vi "PIPBOY_Dlg_MainUi.vi"(11 "Path":path) -> ()   [LabVIEW 2014]
uses:
  PIPBOY_Ctl_Td_PaletteItem.ctl
  <vilib>/picture/picture.llb/imagedata.ctl
  <userlib>/_saphir_lib_vbx.llb/XXX_Tlk_Tree-GetItemPosition_Scalar__saphir_lib_vbx.vi
  <userlib>/_saphir_lib_vbx.llb/XXX_Tlk_Tree-Cleanup_Scalar__saphir_lib_vbx.vi
  <userlib>/_saphir_lib_vbx.llb/XXX_Tlk_Tree-AddElement_Scalar__saphir_lib_vbx.vi
panel:
  in  "ListRemove":bool
  in  "ListAdd":bool
  out "Item Icon":picture
  in  "Item Name":string
  in  "Item Function":i32(ring) items=["<Palette>"=-1, "Complex To Re/Im"=0, "Complex To Polar"=1, "Re/Im To Complex"=2, "Polar To Complex"=3, "Complex Conjugate"=4, "Sign"=5, "Add"=6, "Subtract"=7, "Multiply"=8, "Divide"=9, "Absolute Value"=10, "Round To Nearest"=11, "Quotient & Remainder"=12, "Increment"=13, "Decrement"=14, "Reciprocal"=15, "Square Root"=16, "And"=17, "Or"=18, "Exclusive Or"=19, "Not"=20, "Negate"=21, "Random Number (0-1)"=22, "Not And"=23, "Not Or"=24, "Not Exclusive Or"=25, "Scale By Power Of 2"=26, "Round Toward -Infinity"=27, "Round Toward +Infinity"=28, "Path To String"=29, "String To Path"=30, "Cast Unit Bases"=31, "Implies"=32, "Logical Shift"=33, "Rotate"=34, "First Call?"=35, "DataSocket Open"=36, "DataSocket Close"=37, "DataSocket Read"=38, "DataSocket Write"=39, "Equal?"=40, "Greater Or Equal?"=41, "Less Or Equal?"=42, "Not Equal?"=43, "Max & Min"=44, "Greater?"=45, "Less?"=46, "Empty String/Path?"=47, "Equal To 0?"=48, "Greater Or Equal To 0?"=49, "Less Or Equal To 0?"=50, "Not Equal To 0?"=51, "Greater Than 0?"=52, "Less Than 0?"=53, "Decimal Digit?"=54, "Sort 1D Array"=55, "Hex Digit?"=56, "Printable?"=57, "White Space?"=58, "Lexical Class"=59, "In Range and Coerce"=60, "Not A Number/Path/Refnum?"=61, "Octal Digit?"=62, "To Byte Integer"=63, "To Word Integer"=64, "To Long Integer"=65, "To Unsigned Byte Integer"=66, "To Unsigned Word Integer"=67, "To Unsigned Long Integer"=68, "To Single Precision Float"=69, "To Double Precision Float"=70, "To Extended Precision Float"=71, "Mantissa & Exponent"=72, "To Single Precision Complex"=73, "To Double Precision Complex"=74, "To Extended Precision Complex"=75, "To Quad Integer"=76, "To Unsigned Quad Integer"=77, "Flatten To String"=78, "Unflatten From String"=79, "Swap Bytes"=80, "Swap Words"=81, "Type Cast"=82, "Boolean To (0,1)"=83, "Array To Cluster"=84, "Cluster To Array"=85, "Split Number"=86, "Join Numbers"=87, "Number To Decimal String"=88, "Number To Hexadecimal String"=89, "Number To Octal String"=90, "Number To Engineering String"=91, "Decimal String To Number"=92, "Hexadecimal String To Number"=93, "Octal String To Number"=94, "Fract/Exp String To Number"=95, "To Upper Case"=96, "To Lower Case"=97, "Sine"=98, "Cosine"=99, "Tangent"=100, "Secant"=101, "Cosecant"=102, "Cotangent"=103, "Inverse Sine"=104, "Inverse Cosine"=105, "Inverse Tangent"=106, "Natural Logarithm"=107, "Logarithm Base 10"=108, "Exponential"=109, "Power Of 10"=110, "Power Of X"=111, "Hyperbolic Sine"=112, "Hyperbolic Cosine"=113, "Hyperbolic Tangent"=114, "Inverse Hyperbolic Sine"=115, "Inverse Hyperbolic Cosine"=116, "Inverse Hyperbolic Tangent"=117, "Sine & Cosine"=118, "Natural Logarithm (Arg +1)"=119, "Exponential (Arg) -1"=120, "Power Of 2"=121, "Logarithm Base X"=122, "Logarithm Base 2"=123, "Sinc"=124, "Inverse Tangent (2 Input)"=125, "Tick Count (ms)"=126, "Wait (ms)"=127, "Get Date/Time In Seconds"=128, "Date/Time To Seconds"=129, "Seconds To Date/Time"=130, "Wait Until Next ms Multiple"=131, "Wait For Front Panel Activity"=132, "Generate Front Panel Activity"=133, "One Button Dialog"=134, "Two Button Dialog"=135, "Stop"=136, "Quit LabVIEW"=137, "Control Help Window"=138, "Get Help Window Status"=139, "Control Online Help"=140, "New Directory"=141, "Open File"=142, "New File"=143, "Close File (deprecated)"=144, "Flush File (deprecated)"=145, "Read File"=146, "Write File"=147, "Seek"=148, "EOF"=149, "Lock Range"=150, "Access Rights"=151, "File/Directory Info (deprecated)"=152, "Volume Info"=153, "Move (deprecated)"=154, "Copy (deprecated)"=155, "Delete (deprecated)"=156, "List Directory"=157, "Build Path"=158, "Strip Path"=159, "Path Type"=160, "Array of Strings to Path"=161, "Path to Array of Strings"=162, "Refnum to Path"=163, "VI Library"=164, "Current VI's Path"=165, "Default Directory"=166, "Type and Creator"=167, "Temporary Directory"=168, "String Length"=169, "String Subset"=170, "Number To Exponential String"=171, "Number To Fractional String"=172, "Pick Line"=173, "Append True/False String"=174, "Format Value"=175, "Select"=176, "Index String Array"=177, "Match First String"=178, "Match True/False String"=179, "Scan Value"=180, "Match Pattern"=181, "Rotate String"=182, "Reverse String"=183, "Search/Split String"=184, "Spreadsheet String To Array"=185, "Array To Spreadsheet String"=186, "Get Date/Time String"=187, "Rotate Left With Carry"=188, "Rotate Right With Carry"=189, "String To Byte Array"=190, "Byte Array To String"=191, "Request Deallocation"=192, "Generate Occurrence"=193, "Wait on Occurrence"=194, "Set Occurrence"=195, "IP To String"=196, "String To IP"=197, "TCP Wait On Listener"=198, "TCP Close Connection"=199, "TCP Write"=200, "TCP Open Connection"=201, "TCP Read"=202, "TCP Create Listener"=203, "UDP Open"=204, "UDP Read"=205, "UDP Write"=206, "UDP Close"=207, "Array Size"=208, "Number To Boolean Array"=209, "Boolean Array To Number"=210, "Reverse 1D Array"=211, "Search 1D Array"=212, "Transpose 2D Array"=213, "Add Array Elements"=214, "Multiply Array Elements"=215, "Interpolate 1D Array"=216, "Rotate 1D Array"=217, "Array Max & Min"=218, "Split 1D Array"=219, "Threshold 1D Array"=220, "Or Array Elements"=221, "And Array Elements"=222, "Property Node"=223, "VISA Close"=224, "VISA Find Resource"=225, "VISA Status Description"=226, "VISA Read"=227, "VISA Write"=228, "VISA Clear"=229, "VISA Read STB"=230, "VISA Assert Trigger"=231, "VISA In 16"=232, "VISA Out 16"=233, "VISA Map Address"=234, "VISA Unmap Address"=235, "VISA Peek 16"=236, "VISA Poke 16"=237, "VISA In 8"=238, "VISA Out 8"=239, "VISA Peek 8"=240, "VISA Poke 8"=241, "VISA Disable Event"=242, "VISA Discard Events"=243, "VISA Enable Event"=244, "VISA Wait on Event"=245, "VISA In 32"=246, "VISA Out 32"=247, "VISA Move In 8"=248, "VISA Move Out 8"=249, "VISA Move In 16"=250, "VISA Move Out 16"=251, "GPIB Write"=252, "GPIB Read"=253, "Wait for GPIB RQS"=254, "GPIB Trigger"=255, "GPIB Clear"=256, "GPIB Serial Poll"=257, "GPIB Misc"=258, "GPIB Initialization"=259, "GPIB Wait"=260, "GPIB Status"=261, "AllSpoll"=262, "DevClear"=263, "DevClearList"=264, "EnableLocal"=265, "EnableRemote"=266, "FindLstn"=267, "FindRQS"=268, "MakeAddr"=269, "PassControl"=270, "PPoll"=271, "PPollConfig"=272, "PPollUnconfig"=273, "RcvRespMsg"=274, "ReadStatus"=275, "Receive"=276, "ReceiveSetup"=277, "ResetSys"=278, "Send"=279, "SendCmds"=280, "SendDataBytes"=281, "SendIFC"=282, "SendList"=283, "SendLLO"=284, "SendSetup"=285, "SetRWLS"=286, "SetTimeOut"=287, "TestSRQ"=288, "TestSys"=289, "Trigger"=290, "TriggerList"=291, "WaitSRQ"=292, "VISA Move In 32"=293, "VISA Move Out 32"=294, "VISA Unlock"=295, "VISA Peek 32"=296, "VISA Poke 32"=297, "VISA Memory Allocation"=298, "VISA Memory Free"=299, "Call Chain"=300, "Stacked Sequence Structure"=301, "Case Structure"=302, "For Loop"=303, "1"=304, "Formula Node"=305, "Numeric Constant"=306, "False Constant"=307, "String Constant"=308, "Text Ring (block diagram constant)"=309, "Path Constant"=310, "TDMS Write"=311, "TDMS Read"=312, "TDMS Open"=313, "TDMS Close"=314, "TDMS Set Properties"=315, "TDMS Get Properties"=316, "TDMS List Contents"=317, "TDMS Flush"=318, "Fixed Constant"=319, "TDMS Defragment"=320, "TDMS Advanced Open"=321, "TDMS Set Channel Information"=322, "TDMS Reserve File Size"=323, "TDMS Configure Asynchronous Writes"=324, "TDMS Set Next Write Position"=325, "TDMS Advanced Synchronous Write"=326, "TDMS Configure Asynchronous Reads"=327, "TDMS Start Asynchronous Reads"=328, "TDMS Advanced Read"=329, "TDMS Stop Asynchronous Reads"=330, "TDMS Get Asynchronous Write Status"=331, "TDMS Advanced Close"=332, "TDMS Set Next Read Position"=333, "TDMS Get Asynchronous Read Status"=334, "TDMS Advanced Asynchronous Write"=335, "Listbox Symbol Ring Constant"=336, "Error Ring Constant"=337, "Concatenate Strings"=338, "Build Array"=339, "Index Array"=340, "Array Subset"=341, "Interleave 1D Arrays"=342, "Decimate 1D Array"=343, "Build Cluster Array"=344, "Unbundle"=345, "Bundle"=346, "Code Interface Node"=347, "Event Structure"=348, "Initialize Array"=349, "Diagram Disable Structure"=350, "Reshape Array"=351, "Index & Bundle Cluster Array"=352, "Bundle By Name"=353, "Unbundle By Name"=354, "Convert Unit"=355, "Global Variable"=356, "Local Variable"=357, "Call Library Function Node"=358, "Conditional Disable Structure"=359, "Register For Events"=360, "Build Waveform"=361, "Get Waveform Components"=362, "Time Stamp (block diagram constant)"=363, "Flat Sequence Structure"=364, "Array (block diagram constant)"=365, "Cluster Constant"=366, "ActiveX Container"=367, "Create User Event"=368, "Generate User Event"=369, "Destroy User Event"=370, "Unregister For Events"=371, "Register Event Callback"=372, "Scan From String"=373, "Format Into String"=374, "Scan From File"=375, "Format Into File"=376, "Static VI Reference"=377, "VISA USB Control In"=378, "VISA USB Control Out"=379, "Enum Constant"=380, "VI Server Reference"=381, "Class Specifier Constant"=382, "Knob (modern)"=383, "Push Button"=384, "Rocker"=385, "Numeric Control (modern)"=386, "Numeric Indicator (modern)"=387, "Vertical Toggle Switch (modern)"=388, "Tank (modern)"=389, "Thermometer (modern)"=390, "Meter (modern)"=391, "Gauge (modern)"=392, "Slide Switch"=393, "Round LED (modern)"=394, "Square LED (modern)"=395, "Vertical Fill Slide (modern)"=396, "Text Button"=397, "Vertical Pointer Slide (modern)"=398, "Framed Color Box (modern)"=399, "Horizontal Fill Slide (modern)"=400, "Horizontal Pointer Slide (modern)"=401, "Horizontal Progress Bar (modern)"=402, "Vertical Progress Bar (modern)"=403, "Horizontal Graduated Bar"=404, "Vertical Graduated Bar"=405, "Horizontal Scrollbar"=406, "Vertical Scrollbar"=407, "Simple String"=408, "Color Box Constant"=409, "Listbox"=410, "Table"=411, "Digital Data (modern)"=412, "Stop Button"=413, ".NET Container"=414, "Mixed Checkbox (system)"=415, "VISA In 64"=416, "VISA Out 64"=417, "VISA Peek 64"=418, "VISA Poke 64"=419, "VISA Move In 64"=420, "VISA Move Out 64"=421, "VISA Memory Allocation Ex"=422, "Merge Errors"=423, "Menu Ring (modern)"=424, "Text Ring (modern)"=425, "Pict Ring (modern)"=426, "Text & Pict Ring (modern)"=427, "Combo Box (modern)"=428, "Enum (modern)"=429, "Cluster (modern)"=430, "Array (modern)"=431, "Horizontal Toggle Switch (modern)"=432, "String Control (modern)"=433, "String Indicator (modern)"=434, "Waveform Graph (modern)"=435, "XY Graph (modern)"=436, "Waveform Chart (modern)"=437, "Digital Waveform Graph (modern)"=438, "Intensity Chart (modern)"=439, "Intensity Graph (modern)"=440, "Mixed Signal Graph"=441, "File Path Control (modern)"=442, "File Path Indicator (modern)"=443, "Dial (modern)"=444, "Traditional DAQ Channel (modern)"=445, "IVI Logical Name (modern)"=446, "VISA resource name (modern)"=447, "OK Button (modern)"=448, "Cancel Button (modern)"=449, "Vert Rocker"=450, "Vertical Slide Switch (modern)"=451, "DAQmx Global Channel (modern)"=452, "DAQmx Device Name (modern)"=453, "DAQmx Scale Name (modern)"=454, "DAQmx Switch (modern)"=455, "DAQmx Physical Channel (modern)"=456, "DAQmx Task Name (modern)"=457, "DAQmx Terminal (modern)"=458, "FieldPoint IO Point (modern)"=459, "Motion Resource (modern)"=460, "Table (modern)"=461, "Multicolumn Listbox (modern)"=462, "Listbox (modern)"=463, "Tree (modern)"=464, "Tree (system)"=465, "Table (classic)"=466, "Table (system)"=467, "Multicolumn Listbox (system)"=468, "Multicolumn Listbox (classic)"=469, "Listbox (system)"=470, "Listbox (classic)"=471, "SubPanel"=472, "SubPanel (Classic)"=473, "Shared Variable Control (modern)"=474, "Tree (classic)"=475, "SubPanel (System)"=476, "Vertical Splitter Bar"=477, "Horizontal Splitter Bar"=478, "Vertical Splitter Bar (Classic)"=479, "Horizontal Splitter Bar (Classic)"=480, "Vertical Splitter Bar (System)"=481, "Horizontal Splitter Bar (System)"=482, "Spin Control (system)"=483, "Vertical Pointer Slide (system)"=484, "Horizontal Pointer Slide (system)"=485, "Vertical Slide (system)"=486, "Horizontal Slide (system)"=487, "Vertical Progress Bar (system)"=488, "Horizontal Progress Bar (system)"=489, "Time Stamp Control (modern)"=490, "Time Stamp Indicator (modern)"=491, "Combo Box (system)"=492, "Numeric Control (system)"=493, "String Control (system)"=494, "File Path Control (system)"=495, "Label (modern)"=496, "Label (system)"=497, "Radio Buttons (modern)"=498, "Radio Buttons (system)"=499, "Radio Buttons (classic)"=500, "Compound Arithmetic"=501, "Expression Node"=502, "VISA Set I/O Buffer Size"=503, "VISA Flush I/O Buffer"=504, "VISA Move"=505, "VISA GPIB Control REN"=506, "Inverse Cosecant"=507, "Inverse Secant"=508, "Inverse Cotangent"=509, "Hyperbolic Cosecant"=510, "Hyperbolic Secant"=511, "Hyperbolic Cotangent"=512, "Inverse Hyperbolic Cosecant"=513, "Inverse Hyperbolic Secant"=514, "Inverse Hyperbolic Cotangent"=515, "Square"=516, "VISA VXI Cmd or Query"=517, "Re/Im To Polar"=518, "Polar To Re/Im"=519, "Y-th Root of X"=520, "Empty Array?"=521, "VISA Open"=522, "VISA Assert Interrupt Signal"=523, "VISA Assert Utility Signal"=524, "VISA Map Trigger"=525, "VISA Unmap Trigger"=526, "VISA Read To File"=527, "VISA Write From File"=528, "VISA GPIB Command"=529, "VISA GPIB Control ATN"=530, "VISA GPIB Pass Control"=531, "VISA GPIB Send IFC"=532, "Free Label"=533, "Carriage Return Constant"=534, "Line Feed Constant"=535, "Tab Constant"=536, "Empty String Constant"=537, "Pi"=538, "Pi Multiplied By 2"=539, "Pi Divided By 2"=540, "Reciprocal Of Pi"=541, "Natural Logarithm Of Pi"=542, "Negative Infinity"=543, "Merge Signals"=544, "Natural Logarithm Base"=545, "Reciprocal Of e"=546, "Base 10 Logarithm Of e"=547, "Natural Logarithm Of 10"=548, "Natural Logarithm Of 2"=549, "Positive Infinity"=550, "Planck's Constant (J/Hz)"=551, "Elementary Charge (C)"=552, "Speed Of Light In Vacuum (m/sec)"=553, "Gravitational Constant (N m2/kg2)"=554, "Split Signals"=555, "Avogadro Constant (1/mol)"=556, "Rydberg Constant (1/m)"=557, "Molar Gas Constant (J/(mol K))"=558, "Empty Path Constant"=559, "Not A Path Constant"=560, "End of Line Constant"=561, "Not a Refnum Constant"=562, "Machine Epsilon"=563, "2"=564, "Feedback Node"=565, "Call Parent Method"=566, "MathScript Node"=567, "In Place Element Structure"=568, "3D Picture"=569, "Shared Variable"=570, "Open Variable Connection"=571, "Read Variable"=572, "Write Variable"=573, "Close Variable Connection"=574, "Scanned Variable Read"=575, "Direct Variable Read"=576, "Read Variable with Timeout"=577, "Scanned Variable Write"=578, "Direct Variable Write"=579, "Open and Verify Variable Connection"=580, "Open Variable Connection in Background"=581, "Destroy Stream Endpoint"=582, "Read Single Element from Stream"=583, "Write Single Element to Stream"=584, "Search Variable Container"=585, "Read Multiple Elements from Stream"=586, "Write Multiple Elements to Stream"=587, "Flush Stream"=588, "Create Network Stream Writer Endpoint"=589, "Create Network Stream Reader Endpoint"=590, "Always Copy"=591, "Swap Values"=592, "New Data Value Reference"=593, "Delete Data Value Reference"=594, "CPU Information"=595, "Data Cache Size"=596, "Number of Cache Levels"=597, "Simple Numeric"=598, "Numeric Control (classic)"=599, "Numeric Indicator (classic)"=600, "Simple Vertical Slide"=601, "Simple Horizontal Slide"=602, "Vertical Slide"=603, "Knob (classic)"=604, "Vertical Pointer Slide (classic)"=605, "Framed Color Box (classic)"=606, "Vertical Fill Slide (classic)"=607, "Horizontal Slide (classic)"=608, "Horizontal Pointer Slide (classic)"=609, "Horizontal Fill Slide (classic)"=610, "Color Box"=611, "Text Ring (classic)"=612, "Pict Ring (classic)"=613, "Text & Pict Ring (classic)"=614, "Menu Ring (classic)"=615, "Tank (classic)"=616, "Thermometer (classic)"=617, "Color Ramp"=618, "Enum (classic)"=619, "Meter (classic)"=620, "Gauge (classic)"=621, "Dial (classic)"=622, "Text Ring (system)"=623, "Enum (system)"=624, "Round Button"=625, "Square Button"=626, "Flat Round Button"=627, "Flat Square Button"=628, "Round Light"=629, "Square Light"=630, "Round Radio Button"=631, "Square Radio Button"=632, "Horizontal Switch"=633, "Vertical Switch"=634, "Horizontal Toggle Switch (classic)"=635, "Vertical Toggle Switch (classic)"=636, "Round Push Button (profile)"=637, "Square Push Button (profile)"=638, "Horizontal Slide Switch"=639, "Vertical Slide Switch (classic)"=640, "LED Button"=641, "Checkbox (classic)"=642, "Round Push Button"=643, "Square Push Button"=644, "Round LED (classic)"=645, "Square LED (classic)"=646, "Labeled Round Button"=647, "Labeled Square Button"=648, "Labeled Rectangular Button"=649, "Labeled Oblong Button"=650, "Round Stop Button"=651, "Rectangular Stop Button"=652, "OK Button (system)"=653, "Cancel Button (system)"=654, "Checkbox (system)"=655, "Radio Button (system)"=656, "String Control (classic)"=657, "String Indicator (classic)"=658, "File Path Control (classic)"=659, "File Path Indicator (classic)"=660, "Digital Data (classic)"=661, "Array (classic)"=662, "Combo Box (classic)"=663, "Variant"=664, "DAQmx Scale Name (classic)"=665, "DAQmx Device Name (classic)"=666, "DAQmx Terminal (classic)"=667, "Traditional DAQ Channel (classic)"=668, "Tab Control (classic)"=669, "Tab Control (system)"=670, "Tab Control (modern)"=671, "DAQmx Physical Channel (classic)"=672, "DAQmx Switch (classic)"=673, "Cluster (classic)"=674, "Data Log File Refnum"=675, "Occurrence Refnum"=676, "TCP Network Connection Refnum"=677, "Byte Stream File Refnum"=678, "VISA resource name (classic)"=679, "Automation Refnum"=680, "Application Refnum"=681, "Menu Refnum"=682, "IVI Logical Name (classic)"=683, "IMAQ Session"=684, "DataSocket Refnum"=685, "UDP Network Connection Refnum"=686, "Control Refnum"=687, "IVI Logical Name (block diagram constant)"=688, "VISA Resource Name"=689, "VI Refnum"=690, "Event Callback Refnum"=691, "FieldPoint IO Point (classic)"=692, ".NET Refnum"=693, "DAQmx Task Name (classic)"=694, "DAQmx Global Channel (classic)"=695, "Motion Resource (classic)"=696, "IrDA Network Connection Refnum"=697, "LabVIEW Object"=698, "Bluetooth Network Connection Refnum"=699, "Shared Variable Control (classic)"=700, "XY Graph (classic)"=701, "Waveform Chart (classic)"=702, "Waveform Graph (classic)"=703, "2D Picture"=704, "Intensity Chart (classic)"=705, "Intensity Graph (classic)"=706, "Digital Waveform Graph (classic)"=707, "Raised Box (classic)"=708, "Recessed Box"=709, "Flat Box"=710, "Raised Circle"=711, "Recessed Circle"=712, "Flat Circle"=713, "Raised Frame"=714, "Recessed Frame (modern)"=715, "Flat Frame"=716, "Raised Rounded Box"=717, "Recessed Rounded Box"=718, "Flat Rounded Box"=719, "Raised Left Triangle"=720, "Raised Right Triangle"=721, "Raised Up Triangle"=722, "Raised Down Triangle"=723, "Recessed Left Triangle"=724, "Recessed Right Triangle"=725, "Recessed Up Triangle"=726, "Recessed Down Triangle"=727, "Flat Left Triangle"=728, "Flat Right Triangle"=729, "Flat Up Triangle"=730, "Flat Down Triangle"=731, "Recessed Frame (system)"=732, "Line (thin)"=733, "Line with Arrow (thin)"=734, "Line (thick)"=735, "Line with Arrow (thick)"=736, "Horizontal Smooth Box"=737, "Vertical Smooth Box"=738, "Lowered Box (thick)"=739, "Horizontal Button Box"=740, "Raised Box (modern)"=741, "Lowered Rounded Box"=742, "Invoke Node"=743, "Call By Reference Node"=744, "Constructor Node"=745, "Replace Array Subset"=746, "Insert Into Array"=747, "Delete From Array"=748, "Replace Substring"=749, "Search and Replace String"=750, "Select a VI..."=751, "Select a Control..."=752, "Time Stamp Control (classic)"=753, "Time Stamp Indicator (classic)"=754, "To Time Stamp"=755, "To Fixed-Point"=756, "Clear Fixed-Point Overflow Status"=757, "Remove Fixed-Point Overflow Status"=758, "Include Fixed-Point Overflow Status"=759, "Fixed-Point Overflow?"=760, "Fixed-Point to Integer Cast"=761, "Integer to Fixed-Point Cast"=762, "Timed Loop"=763, "Timed Sequence"=764, "Automation Open"=765, "Variant To Data"=766, "Open VI Reference"=767, "Close Reference"=768, "Open Application Reference"=769, "Open VI Object Reference"=770, "New VI"=771, "New VI Object"=772, "To More Specific Class"=773, "To More Generic Class"=774, "Preserve Run-Time Class"=775, "Open/Create/Replace File"=776, "Read from Binary File"=777, "Close File"=778, "Copy"=779, "Open/Create/Replace Datalog"=780, "Create Folder"=781, "Delete"=782, "Deny Access"=783, "Flush File"=784, "Get Datalog Position"=785, "Get File Position"=786, "Get File Size"=787, "Get Number of Records"=788, "Get Permissions"=789, "Get Type and Creator"=790, "Get Volume Info"=791, "Move"=792, "Read Datalog"=793, "Read from Text File"=794, "Set Datalog Position"=795, "Set File Position"=796, "Set File Size"=797, "Set Number of Records"=798, "Set Permissions"=799, "Set Type and Creator"=800, "Write to Binary File"=801, "Write Datalog"=802, "Write to Text File"=803, "File Dialog (deprecated)"=804, "File/Directory Info"=805, "List Folder"=806, "Format Date/Time String"=807, "Scan String For Tokens"=808, "To Variant"=809, "Flattened String To Variant"=810, "Variant To Flattened String"=811, "Set Variant Attribute"=812, "Get Variant Attribute"=813, "Delete Variant Attribute"=814, "Set Waveform Attribute"=815, "Get Waveform Attribute"=816, "Flatten To XML"=817, "Unflatten From XML"=818, "Build Matrix"=819, "Get Matrix Diagonal"=820, "Get Matrix Elements"=821, "Get Submatrix"=822, "Set Matrix Diagonal"=823, "Set Matrix Elements"=824, "Set Submatrix"=825, "Matrix Size"=826, "Resize Matrix"=827, "Transpose Matrix"=828, "Current VI's Menubar"=829, "Get Menu Selection"=830, "Enable Menu Tracking"=831, "Insert Menu Items"=832, "Delete Menu Items"=833, "Get Menu Item Info"=834, "Set Menu Item Info"=835, "Get Menu Short Cut Info"=836, "MATLAB script"=837, "Obtain Notifier"=838, "Release Notifier"=839, "Get Notifier Status"=840, "Send Notification"=841, "Wait on Notification"=842, "Wait on Notification from Multiple"=843, "Cancel Notification"=844, "Obtain Queue"=845, "Release Queue"=846, "Get Queue Status"=847, "Enqueue Element"=848, "Preview Queue Element"=849, "Dequeue Element"=850, "Flush Queue"=851, "Enqueue Element At Opposite End"=852, "Lossy Enqueue Element"=853, "Wait on Notification with Notifier History"=854, "Wait on Notification from Multiple with Notifier History"=855, "IrDA Create Listener"=856, "IrDA Discover"=857, "IrDA Open Connection"=858, "IrDA Wait On Listener"=859, "IrDA Close Connection"=860, "IrDA Read"=861, "IrDA Write"=862, "Bluetooth Wait On Listener"=863, "Bluetooth Close Connection"=864, "Bluetooth Read"=865, "Bluetooth Write"=866, "Bluetooth Create Listener"=867, "Bluetooth Discover"=868, "Bluetooth Open Connection"=869, "Get Drag Drop Data"=870]
  in  "Palettes":string(tree)
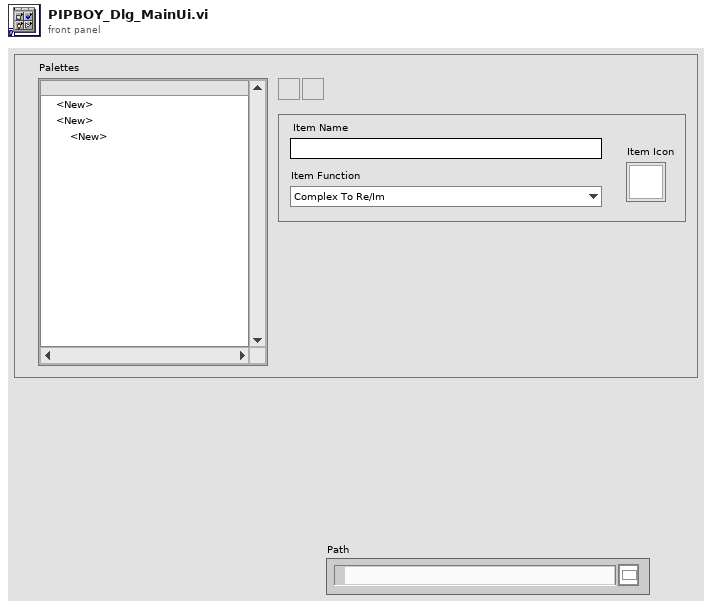
[diagram p1: front panel]
types:
  T1 = typedef "PIPBOY_Ctl_Td_PaletteItem.ctl" = cluster{"Name":string, "Function":string, "Palette(T)/Item(F)":bool, "Icon":T2}
  T2 = typedef "imagedata.ctl" = cluster{"image type":i32, "image depth":i32, "image":u8[], "mask":u8[], "colors":u32[], "Rectangle":cluster{"left":i16, "top":i16, "right":i16, "bottom":i16}}
  T3 = cluster{"ChildLabel":string, "ChildRowDatas":string[]}
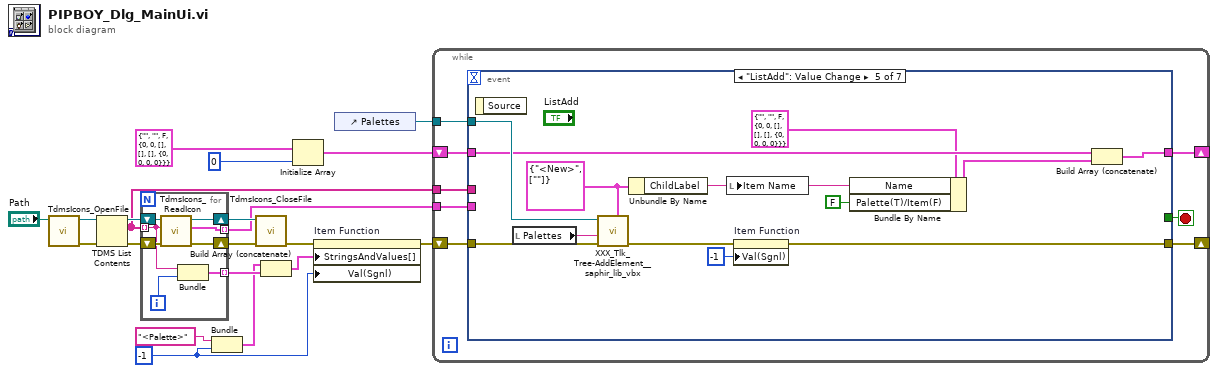
[diagram p0: block diagram]
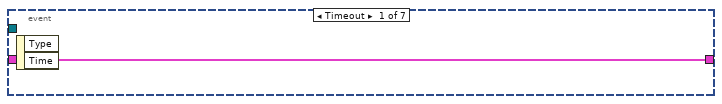
[diagram p2: hidden frame]
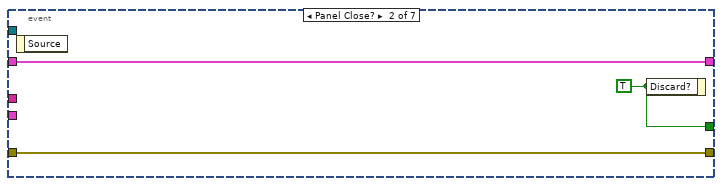
[diagram p3: hidden frame]
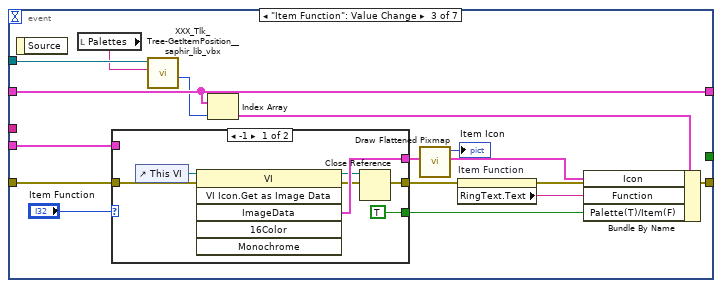
[diagram p4: hidden frame]
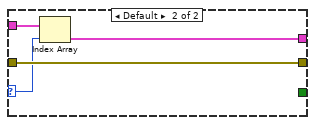
[diagram p5: hidden frame]
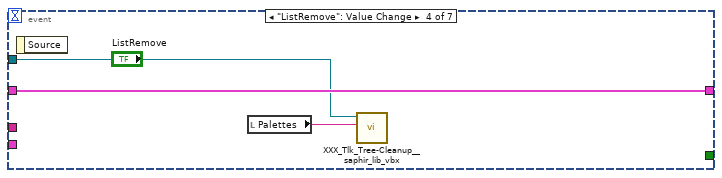
[diagram p6: hidden frame]
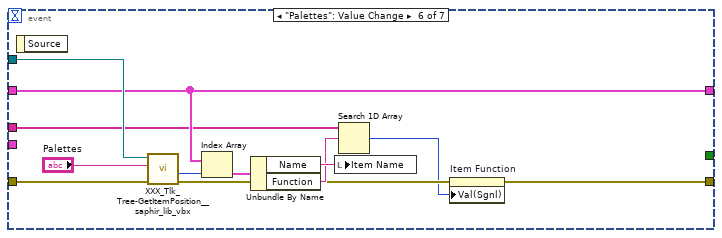
[diagram p7: hidden frame]
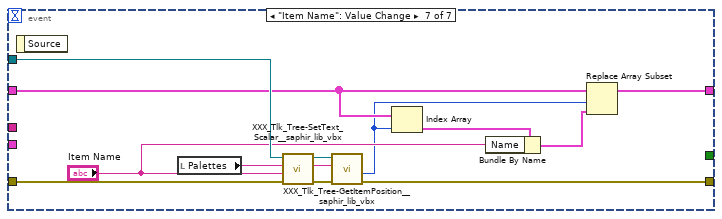
[diagram p8: hidden frame]
diagram:
  w2 = -1
  n1 = call "TdmsIcons_OpenFile.vi"("Path"="Path") -> ("error out"=w17:errorcluster, "TdmsOut"=w13:refnum<k34>)  [unwired: 9 in]
  n2 = TDMS List Contents(4:w17, 7:w13) -> (0:w14:errorcluster, 2:w10:string[], 3:w12:refnum<k34>)  [unwired: 1 in, 1 out]
  n3 = for {
    shift-right: [w28] -> w16
    shift-left: w14 -> [w26]
    shift-right: [w27] -> w15
    shift-left: w12 -> [w25]
    tunnel: w10 -> [w23] mode=indexing
    tunnel: [w24] -> w11 mode=indexing
    tunnel: [w21] -> w9 mode=indexing
    i -> [w22]
    n4 = call "TdmsIcons_ReadIcon.vi"("error in (no error)"=w26, "Function"=w23, "TdmsIn"=w25) -> ("error out"=w28:errorcluster, "Icon"=w24:T2, "TdmsOut"=w27:refnum<k34>)  [unwired: 6 in]
    n5 = Bundle(w23, w22) -> (w21:cluster{string, i32})  [unwired: 1 in]
  }
  n6 = Bundle("<Palette>", w2) -> (w7:cluster{string, i32})  [unwired: 1 in]
  n7 = call "TdmsIcons_CloseFile.vi"("error in (no error)"=w16, "TdmsIn"=w15) -> ("error out"=w6:errorcluster)  [unwired: 8 in, 1 out]
  n8 = Build Array (concatenate)(w7, w9) -> (w4:cluster{string, i32}[])
  n9 = Initialize Array(T1 {"Name"="", "Function"="", "Palette(T)/Item(F)"=FALSE, "Icon"={"image type"=0, "image depth"=0, "image"=[], "mask"=[], "colors"=[], "Rectangle"={"left"=0, "top"=0, "right"=0, "bottom"=0}}} ("Item"), 0 ("dimension size")) -> (w18:T1[])
  n10 = property on="Item Function" class="Ring (strict)"(error in=w6, "StringsAndValues[]"=w4, "Val(Sgnl)"=w2) -> (error out=w5:errorcluster)  [unwired: 1 in, 1 out]
  n11 = control-ref of="Palettes"() -> (w1:refnum<vi>)
  n12 = while {
    shift-right: [w34] -> _
    shift-left: w18 -> [w35]
    shift-right: [w32] -> _
    shift-left: w5 -> [w33]
    tunnel: w11 -> [w31]
    tunnel: w10 -> [w29]
    tunnel: w1 -> [w30]
    stop <- w36 stop-if-true
    n13 = event shown="[4] \"ListAdd\": Value Change" {
      selector: _ -> [_ _ _ _ _ _ _]
      dyn-events: _ -> [_ _ _ _ _ _ _]
      timeout: _ -> [_ _ _ _ _ _ _]
      tunnel: [_ w40 _ _ _ _ _] -> w36
      tunnel: w35 -> [w37 w39 w46 w67 w78 w89 w96]
      tunnel: [w37 w39 w46 w67 w77 w89 w95] -> w34
      tunnel: w33 -> [_ w38 w51 _ w80 w92 w100]
      tunnel: [_ w38 w49 _ w73 w82 w99] -> w32
      tunnel: w31 -> [_ _ w54 _ _ _ _]
      tunnel: w30 -> [_ _ w48 w66 w79 w91 w105]
      tunnel: w29 -> [_ _ _ _ _ w85 _]
      event Timeout {
        n14 = event-data() -> ()  [unwired: 3 out]
      }
      event Panel Close? {
        w40 = TRUE ("Discard?")
        n15 = event-data() -> ()  [unwired: 2 out]
        n16 = event-data("Discard?"=w40) -> ()  [unwired: 1 in, 1 out]
      }
      event "Item Function": Value Change {
        n17 = event-data() -> ()  [unwired: 2 out]
        n18 = local read "Palettes"() -> (w47:string)
        n19 = case shown="-1" "Item Function" {
          selector: "Item Function" -> [_ w61]
          tunnel: w54 -> [_ w64]
          tunnel: [w58 w63] -> w41
          tunnel: w51 -> [w59 w62]
          tunnel: [w57 w62] -> w50
          tunnel: [TRUE _] -> w42
          frame -1 {
            n20 = control-ref of="This VI"() -> (w60:refnum<vi>)
            n21 = invoke class="VI" method="VI Icon.Get as Image Data"(reference=w60, error in=w59) -> (reference out=w56:refnum<vi>, error out=w57:errorcluster, "ImageData"=w58:T2)  [unwired: 4 in, 3 out]
            n22 = Close Reference(reference=w56) -> ()  [unwired: 1 in, 1 out]
          }
          frame Default {
            n23 = Index Array(array=w64, index=w61) -> (element=w63:T2)
          }
        }
        n24 = call-poly <userlib>:"XXX_Tlk_Tree-GetItemPosition__saphir_lib_vbx.vi"("ElementTag"=w47, "TreeRefNum"=w48) -> ("Position"=w45:i32)  [unwired: 6 in, 3 out]
        n25 = Index Array(array=w46, index=w45) -> (element=w44:T1)
        n26 = call <vilib>:"Draw Flattened Pixmap.vi"("image data"=w41) -> ("new picture"=→"Item Icon":picture)  [unwired: 8 in]
        n27 = property on="Item Function" class="Ring (strict)"(error in=w50) -> (error out=w49:errorcluster, "RingText.Text"=w43:string)  [unwired: 1 in, 1 out]
        n28 = Bundle By Name(cluster=w44, "Icon"=w41, "Function"=w43, "Palette(T)/Item(F)"=w42) -> ()  [unwired: 1 out]
      }
      event "ListRemove": Value Change {
        n29 = event-data() -> ()  [unwired: 2 out]
        n30 = local read "Palettes"() -> (w65:string)
        n31 = call-poly <userlib>:"XXX_Tlk_Tree-Cleanup__saphir_lib_vbx.vi"("ElementTag"=w65, "TreeRefNum"=w66) -> ()  [unwired: 8 in, 2 out]
      }
      event "ListAdd": Value Change {
        w76 = T3 {"ChildLabel"="<New>", "ChildRowDatas"=[""]} ("ChildProperty")
        n32 = event-data() -> ()  [unwired: 2 out]
        n33 = local read "Palettes"() -> (w68:string)
        n34 = call-poly <userlib>:"XXX_Tlk_Tree-AddElement__saphir_lib_vbx.vi"("ChildProperty"=w76, "error in"=w80, "ParentTag (empty)"=w68, "TreeRefNum"=w79) -> ("error out"=w74:errorcluster)  [unwired: 5 in, 2 out]
        n35 = Unbundle By Name(w76) -> ("ChildLabel"=w71:string)
        n36 = local write "Item Name"(w71) -> ()
        n37 = property on="Item Function" class="Ring (strict)"(error in=w74, "Val(Sgnl)"=-1 ("Value (Signaling)")) -> (error out=w73:errorcluster)  [unwired: 1 in, 1 out]
        n38 = Bundle By Name(cluster=T1 {"Name"="", "Function"="", "Palette(T)/Item(F)"=FALSE, "Icon"={"image type"=0, "image depth"=0, "image"=[], "mask"=[], "colors"=[], "Rectangle"={"left"=0, "top"=0, "right"=0, "bottom"=0}}} ("Item"), "Name"=w71, "Palette(T)/Item(F)"=FALSE) -> (w70:T1)
        n39 = Build Array (concatenate)(w78, w70) -> (w77:T1[])
      }
      event "Palettes": Value Change {
        n40 = event-data() -> ()  [unwired: 2 out]
        n41 = call-poly <userlib>:"XXX_Tlk_Tree-GetItemPosition__saphir_lib_vbx.vi"("error in"=w92, "ElementTag"="Palettes", "TreeRefNum"=w91) -> ("error out"=w83:errorcluster, "Position"=w88:i32)  [unwired: 5 in, 2 out]
        n42 = Index Array(array=w89, index=w88) -> (element=w87:T1)
        n43 = Unbundle By Name(w87) -> ("Name"=w86:string, "Function"=w84:string)
        n44 = local write "Item Name"(w86) -> ()
        n45 = Search 1D Array(1D array=w85, element=w84) -> (index of element=w81:i32)  [unwired: 1 in]
        n46 = property on="Item Function" class="Ring (strict)"(error in=w83, "Val(Sgnl)"=w81) -> (error out=w82:errorcluster)  [unwired: 1 in, 1 out]
      }
      event "Item Name": Value Change {
        n47 = event-data() -> ()  [unwired: 2 out]
        n48 = local read "Palettes"() -> (w104:string)
        n49 = call <userlib>:"XXX_Tlk_Tree-SetText_Scalar__saphir_lib_vbx.vi"("error in (no error)"=w100, "CellString"="Item Name", "ElementTag"=w104, "TreeRefNum"=w105) -> ("error out"=w101:errorcluster, "ElementTagDuplicated"=w102:string, "TreeRefNumDuplicated"=w103:refnum<vi>)  [unwired: 4 in, 1 out]
        n50 = call-poly <userlib>:"XXX_Tlk_Tree-GetItemPosition__saphir_lib_vbx.vi"("error in"=w101, "ElementTag"=w102, "TreeRefNum"=w103) -> ("error out"=w99:errorcluster, "Position"=w93:i32)  [unwired: 5 in, 2 out]
        n51 = Index Array(array=w96, index=w93) -> (element=w98:T1)
        n52 = Bundle By Name(cluster=w98, "Name"="Item Name") -> (w94:T1)
        n53 = Replace Array Subset(array=w96, new element=w94, index=w93) -> (w95:T1[])
      }
    }
  }
